vi "Create.vi"(8 "error in (no error)":errorcluster, 10 "config file path":path, 11 "BASE in":refnum<class "BASE.lvclass">) -> (0 "error out":errorcluster, 2 "Actor's Enqueuer":refnum<class "Message Enqueuer.lvclass">, 3 "BASE out":refnum<class "BASE.lvclass">)   [LabVIEW 2019, in "BASE.lvlib" / "BASE.lvclass"]
uses:
  BASE.lvclass
  D:/Program Files (x86)/National Instruments/LabVIEW 2019/vi.lib/ActorFramework/Actor/Actor.lvclass
  <vilib>/ActorFramework/Message Enqueuer/Message Enqueuer.lvclass
  <vilib>/ActorFramework/Actor/Actor.lvclass
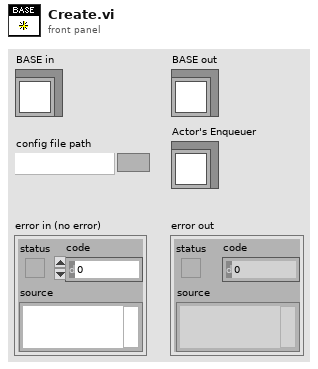
[diagram p1: front panel]
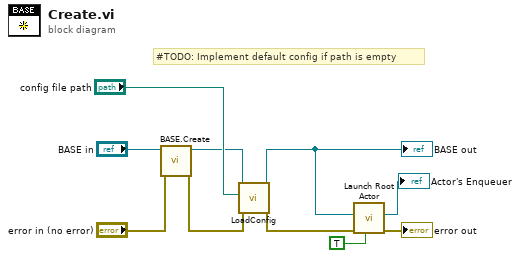
[diagram p0: block diagram]
diagram:
  # "#TODO: Implement default config if path is empty"
  n1 = call-dynamic "BASE.Create.vi"("error in (no error)"="error in (no error)", "BASE in"="BASE in") -> ("error out"=w1:errorcluster, "BASE out"=w3:refnum<class "BASE.lvclass">)  [unwired: 8 in]
  n2 = call "LoadConfig.vi"("error in (no error)"=w1, "config file path (Empty: use configured)"="config file path", "BASE in"=w3) -> ("error out"=w7:errorcluster, "BASE out"=w5:refnum<class "BASE.lvclass">)  [unwired: 7 in]
  "BASE out" <- w5
  n3 = call <vilib>:"Launch Root Actor.vi"("Open Actor Core front panel? (F)"=TRUE, "error in (no error)"=w7, "Actor"=w5) -> ("error out"=→"error out":errorcluster, "Actor's Enqueuer"=→"Actor's Enqueuer":refnum<class "Message Enqueuer.lvclass">)  [unwired: 7 in]
